vi "NT_LL_Write String.vi"(8 "error in (no error)":errorcluster, 9 "value":string, 10 "timestamp":u64, 11 "publishHandle":u32) -> (0 "error out":errorcluster, 3 "success":u32)   [LabVIEW 2025]
uses:
  FRC_NetworkTablesLV.dll
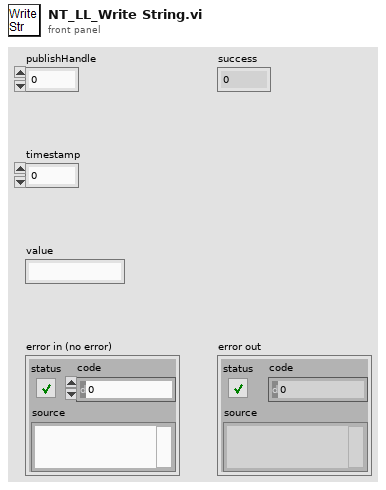
[diagram p1: front panel]
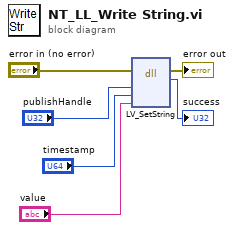
[diagram p0: block diagram]
diagram:
  n1 = dll-call lib="FRC_NetworkTablesLV.*" fn="LV_SetString"(error in="error in (no error)", "publishHandle"="publishHandle", "time"="timestamp", "value"="value") -> (error out=→"error out":errorcluster, "success"=→"success":u32)  [unwired: 5 in, 1 out]
